vi "WLAN - TV - OPPO - RW - ReadTestVectorFile.vi"(5 "TV":string[][](array[string]), 7 "Measure Config":string[][](array[string])) -> (6 "Tv First Element":T2 {"Standard" items=["80211A/G/J/P OFDM", "80211B/G DSSS", "80211G DSSSOFDM", "80211N MIMOOFDM", "80211AC MIMOOFDM"]; "OFDM Data Rate (Mbps)" items=["6", "9", "12", "18", "24", "36", "48", "54"]; "80211n PLCP Frame Format" items=["Mixed Format", "Greenfield Format"]; "FEC Coding Type" items=["BCC", "LDPC"]; "DSSS Data Rate (Mbps)" items=["1", "2", "5.5 CCK", "5.5 PBCC", "11 CCK", "11 PBCC", "22", "33"]}, 10 "WLAN Measurement Settings":T3={"OFDM Advanced Controls(11ag)"={"OFDM Auto Compute Acquisition Length Enabled"=0, "OFDM Maximum Symbols Used"=0, "OFDM Time Tracking Enabled"=0, "OFDM Channel Tracking Enabled"=0, "OFDM Amplitude Tracking Enabled"=1, "OFDM CFO Estimation Method"=0, "OFDM Phase Tracking Method"=0, "OFDM Header Detection Enabled"=0, "OFDM MAC FCS Check Enabled"=0, "#Avg"=10, "#Iterations"=10}, "DSSS Demod Parameters"={"DSSS Auto Compute Acquisition Length Enabled"=0, "DSSS Equalization Enabled"=0, "DSSS Header Detection Enabled"=0, "DSSS MAC FCS Check Enabled"=0, "DSSS Measurement Start Location"=0, "DSSS Phase Tracking Method"=0, "DSSS Maximum Chips Used"=0, "DSSS Reference Pulse Shaping Filter"=0, "DSSS Reference Pulse Shaping Filter Coefficient"=0.0, "# Avg"=1024, "# Iterations"=1024, "DSSS Power Ramp Enabled"=0}, "OFDM Advanced Controls (11n)"={"OFDM Auto Compute Acquisition Length Enabled"=0, "OFDM Maximum Symbols Used"=0, "OFDM Time Tracking Enabled"=0, "OFDM Channel Tracking Enabled"=0, "OFDM Amplitude Tracking Enabled"=1, "OFDM CFO Estimation Method"=0, "OFDM Phase Tracking Method"=0, "OFDM Header Detection Enabled"=0, "OFDM MAC FCS Check Enabled"=0, "#Avg"=10, "#Iterations"=10}, "OFDM Advanced Controls(11ac)"={"OFDM Auto Compute Acquisition Length Enabled"=0, "OFDM Maximum Symbols Used"=0, "OFDM Time Tracking Enabled"=1, "OFDM Channel Tracking Enabled"=0, "OFDM Amplitude Tracking Enabled"=0, "OFDM CFO Estimation Method"=0, "OFDM Phase Tracking Method"=0, "OFDM Header Detection Enabled"=0, "OFDM MAC FCS Check Enabled"=0, "#Avg"=10, "#Iterations"=10}} {"OFDM Advanced Controls(11ac)"."OFDM Phase Tracking Method" items=["Standard", "Instantaneous", "None", "Standard with Cubic Spline Fit"]; "OFDM Advanced Controls(11ac)"."OFDM CFO Estimation Method" items=["Preamble Only", "Preamble and Data"]; "OFDM Advanced Controls(11ac)"."OFDM Channel Tracking Enabled" items=["False", "True"]; "OFDM Advanced Controls(11ac)"."OFDM Amplitude Tracking Enabled" items=["False", "True"]; "OFDM Advanced Controls(11ac)"."OFDM Time Tracking Enabled" items=["True"=1, "False"=0]; "OFDM Advanced Controls(11ac)"."OFDM Auto Compute Acquisition Length Enabled" items=["False", "True"]; "OFDM Advanced Controls(11ac)"."OFDM MAC FCS Check Enabled" items=["False", "True"]; "OFDM Advanced Controls(11ac)"."OFDM Header Detection Enabled" items=["False", "True"]; "OFDM Advanced Controls (11n)"."OFDM Phase Tracking Method" items=["Standard", "Instantaneous", "None", "Standard with Cubic Spline Fit"]; "OFDM Advanced Controls (11n)"."OFDM CFO Estimation Method" items=["Preamble Only", "Preamble and Data"]; "OFDM Advanced Controls (11n)"."OFDM Channel Tracking Enabled" items=["False", "True"]; "OFDM Advanced Controls (11n)"."OFDM Amplitude Tracking Enabled" items=["False", "True"]; "OFDM Advanced Controls (11n)"."OFDM Time Tracking Enabled" items=["True"=1, "False"=0]; "OFDM Advanced Controls (11n)"."OFDM Auto Compute Acquisition Length Enabled" items=["False", "True"]; "OFDM Advanced Controls (11n)"."OFDM MAC FCS Check Enabled" items=["False", "True"]; "OFDM Advanced Controls (11n)"."OFDM Header Detection Enabled" items=["False", "True"]; "DSSS Demod Parameters"."DSSS Power Ramp Enabled" items=["False", "True"]; "DSSS Demod Parameters"."DSSS Auto Compute Acquisition Length Enabled" items=["False", "True"]; "DSSS Demod Parameters"."DSSS Phase Tracking Method" items=["Standard", "Instantaneous"]; "DSSS Demod Parameters"."DSSS Equalization Enabled" items=["False", "True"]; "DSSS Demod Parameters"."DSSS Reference Pulse Shaping Filter" items=["Rectangular", "Raised Cosine", "Root Raised Cosine", "Gaussian"]; "DSSS Demod Parameters"."DSSS MAC FCS Check Enabled" items=["False", "True"]; "DSSS Demod Parameters"."DSSS Header Detection Enabled" items=["False", "True"]; "OFDM Advanced Controls(11ag)"."OFDM Phase Tracking Method" items=["Standard", "Instantaneous", "None", "Standard with Cubic Spline Fit"]; "OFDM Advanced Controls(11ag)"."OFDM CFO Estimation Method" items=["Preamble Only", "Preamble and Data"]; "OFDM Advanced Controls(11ag)"."OFDM Channel Tracking Enabled" items=["False", "True"]; "OFDM Advanced Controls(11ag)"."OFDM Amplitude Tracking Enabled" items=["False", "True"]; "OFDM Advanced Controls(11ag)"."OFDM Time Tracking Enabled" items=["True"=1, "False"=0]; "OFDM Advanced Controls(11ag)"."OFDM Auto Compute Acquisition Length Enabled" items=["False", "True"]; "OFDM Advanced Controls(11ag)"."OFDM MAC FCS Check Enabled" items=["False", "True"]; "OFDM Advanced Controls(11ag)"."OFDM Header Detection Enabled" items=["False", "True"]}, 14 "Cluster":T6)   [LabVIEW 2012]
uses:
  Includes/WLAN - TV - RW - INC - TV_DataType_Cluster.ctl
  Includes/WLAN - TV - RW - INC - Tx_Measurement_Cluster.ctl
  Includes/WLAN - TV - RW - INC - TV_OFDM Demod.ctl
  Includes/WLAN - TV - RW - INC - TV_DSSS Demod.ctl
  Includes/WLAN - TV - RW - INC - Tx_Measurement_Cluster(string).ctl
  Includes/WLAN - TV - RW - INC - Tx_Meas_Settings_OFDM_String.ctl
  Includes/WLAN - TV - RW - INC - Tx_Meas_Settings_DSSS_String.ctl
  Includes/WLAN - TV - RW - INC - TV_Parameters.ctl
panel:
  out "element":string
  in  "Tab Control":T1(tab)
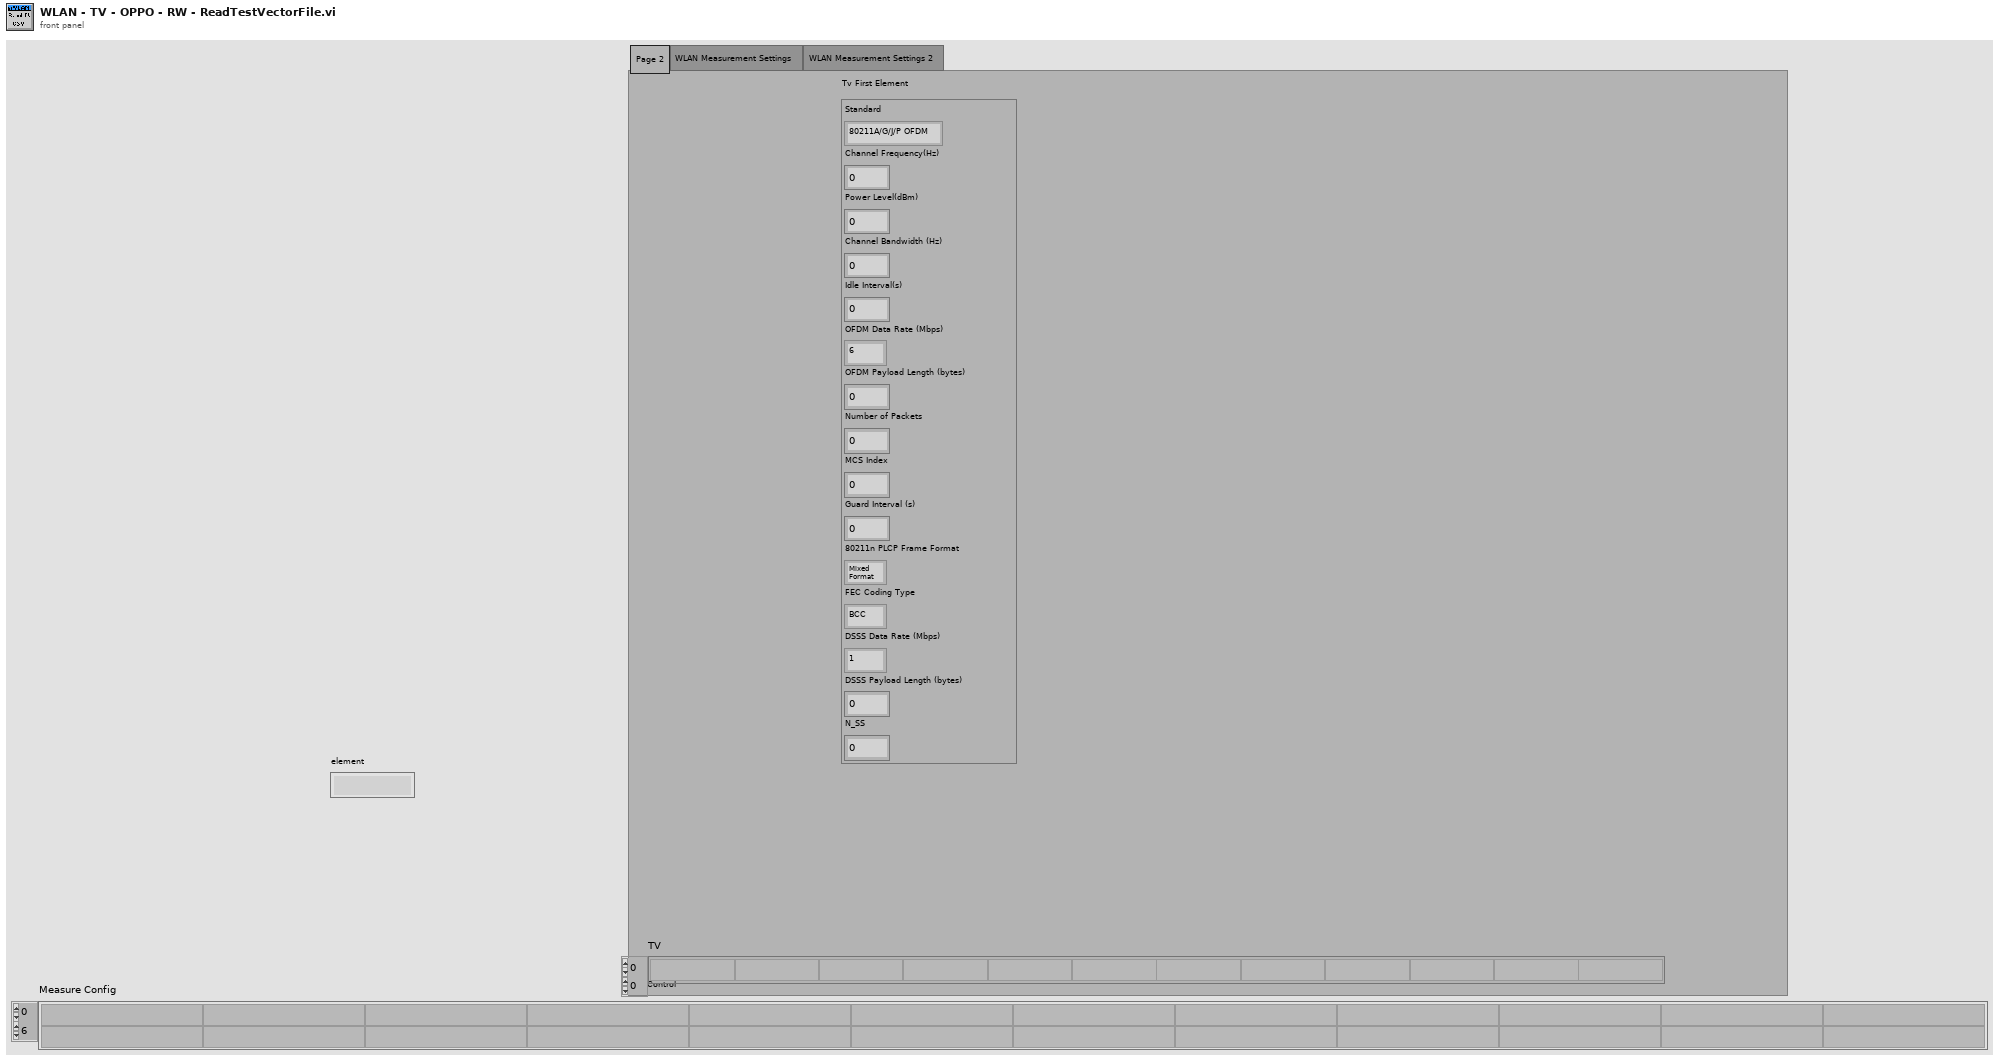
[diagram p1: front panel]
types:
  T1 = enum32{"Page 2", "WLAN Measurement Settings", "WLAN Measurement Settings 2"}
  T2 = typedef "WLAN - TV - RW - INC - TV_DataType_Cluster.ctl" = cluster{"Standard":i32, "Channel Frequency(Hz)":dbl, "Power Level(dBm)":dbl, "Channel Bandwidth (Hz)":dbl, "Idle Interval(s)":dbl, "OFDM Data Rate (Mbps)":i32, "OFDM Payload Length (bytes)":i32, "Number of Packets":i32, "MCS Index":i32, "Guard Interval (s)":dbl, "80211n PLCP Frame Format":i32, "FEC Coding Type":i32, "DSSS Data Rate (Mbps)":i32, "DSSS Payload Length (bytes)":i32, "N_SS":i32}
  T3 = typedef "WLAN - TV - RW - INC - Tx_Measurement_Cluster.ctl" = cluster{"OFDM Advanced Controls(11ag)":T4, "DSSS Demod Parameters":T5, "OFDM Advanced Controls (11n)":T4, "OFDM Advanced Controls(11ac)":cluster{"OFDM Auto Compute Acquisition Length Enabled":i32, "OFDM Maximum Symbols Used":i32, "OFDM Time Tracking Enabled":i32, "OFDM Channel Tracking Enabled":i32, "OFDM Amplitude Tracking Enabled":i32, "OFDM CFO Estimation Method":i32, "OFDM Phase Tracking Method":i32, "OFDM Header Detection Enabled":i32, "OFDM MAC FCS Check Enabled":i32, "#Avg":i32, "#Iterations":i32}}
  T4 = typedef "WLAN - TV - RW - INC - TV_OFDM Demod.ctl" = cluster{"OFDM Auto Compute Acquisition Length Enabled":i32, "OFDM Maximum Symbols Used":i32, "OFDM Time Tracking Enabled":i32, "OFDM Channel Tracking Enabled":i32, "OFDM Amplitude Tracking Enabled":i32, "OFDM CFO Estimation Method":i32, "OFDM Phase Tracking Method":i32, "OFDM Header Detection Enabled":i32, "OFDM MAC FCS Check Enabled":i32, "#Avg":i32, "#Iterations":i32}
  T5 = typedef "WLAN - TV - RW - INC - TV_DSSS Demod.ctl" = cluster{"DSSS Auto Compute Acquisition Length Enabled":i32, "DSSS Equalization Enabled":i32, "DSSS Header Detection Enabled":i32, "DSSS MAC FCS Check Enabled":i32, "DSSS Measurement Start Location":i32, "DSSS Phase Tracking Method":i32, "DSSS Maximum Chips Used":i32, "DSSS Reference Pulse Shaping Filter":i32, "DSSS Reference Pulse Shaping Filter Coefficient":dbl, "# Avg":i32, "# Iterations":i32, "DSSS Power Ramp Enabled":i32}
  T6 = typedef "WLAN - TV - RW - INC - Tx_Measurement_Cluster(string).ctl" = cluster{"OFDM Measurement Settings(11a)":T7, "TV Paramaters(11b)":T8, "OFDM Measurement Settings(11n) ":T7, "OFDM Measurement Settings(11ac) ":T7}
  T7 = typedef "WLAN - TV - RW - INC - Tx_Meas_Settings_OFDM_String.ctl" = cluster{"OFDM Auto Compute Acquisition Length Enabled":string, "OFDM Maximum Symbols Used":string, "OFDM Time Tracking Enabled":string, "OFDM Channel Tracking Enabled":string, "OFDM Amplitude Tracking Enabled":string, "OFDM CFO Estimation Method":string, "OFDM Phase Tracking Method":string, "OFDM Header Detection Enabled":string, "OFDM MAC FCS Check Enabled":string, "#Avg":string, "#Iterations":string}
  T8 = typedef "WLAN - TV - RW - INC - Tx_Meas_Settings_DSSS_String.ctl" = cluster{"DSSS Auto Compute Acquisition Length Enabled":string, "DSSS Equalization Enabled":string, "DSSS Header Detection Enabled":string, "DSSS MAC FCS Check Enabled":string, "DSSS Measurement Start Location":string, "DSSS Phase Tracking Method":string, "DSSS Maximum Chips Used":string, "DSSS Reference Pulse Shaping Filter":string, "DSSS Reference Pulse Shaping Filter Coefficient":string, "#Avg":string, "#Iterations":string, "DSSS Ramp Enabled ":string}
  T9 = typedef "WLAN - TV - RW - INC - TV_Parameters.ctl" = cluster{"Standard ":string, "Channel Frequency(Hz)":string, "Power Level(dBm)":string, "Channel Bandwidth (Hz)":string, "Idle Interval (s)":string, "OFDM Data Rate (Mbps)":string, "OFDM Payload Length (bytes)":string, "MCS Index":string, "Guard Interval (s)":string, "80211n PLCP Frame Format":string, "FEC Coding Type":string, "DSSS Data Rate (Mbps)":string, "DSSS Payload Length (bytes)":string, "#Packets":string, "N_SS":string}
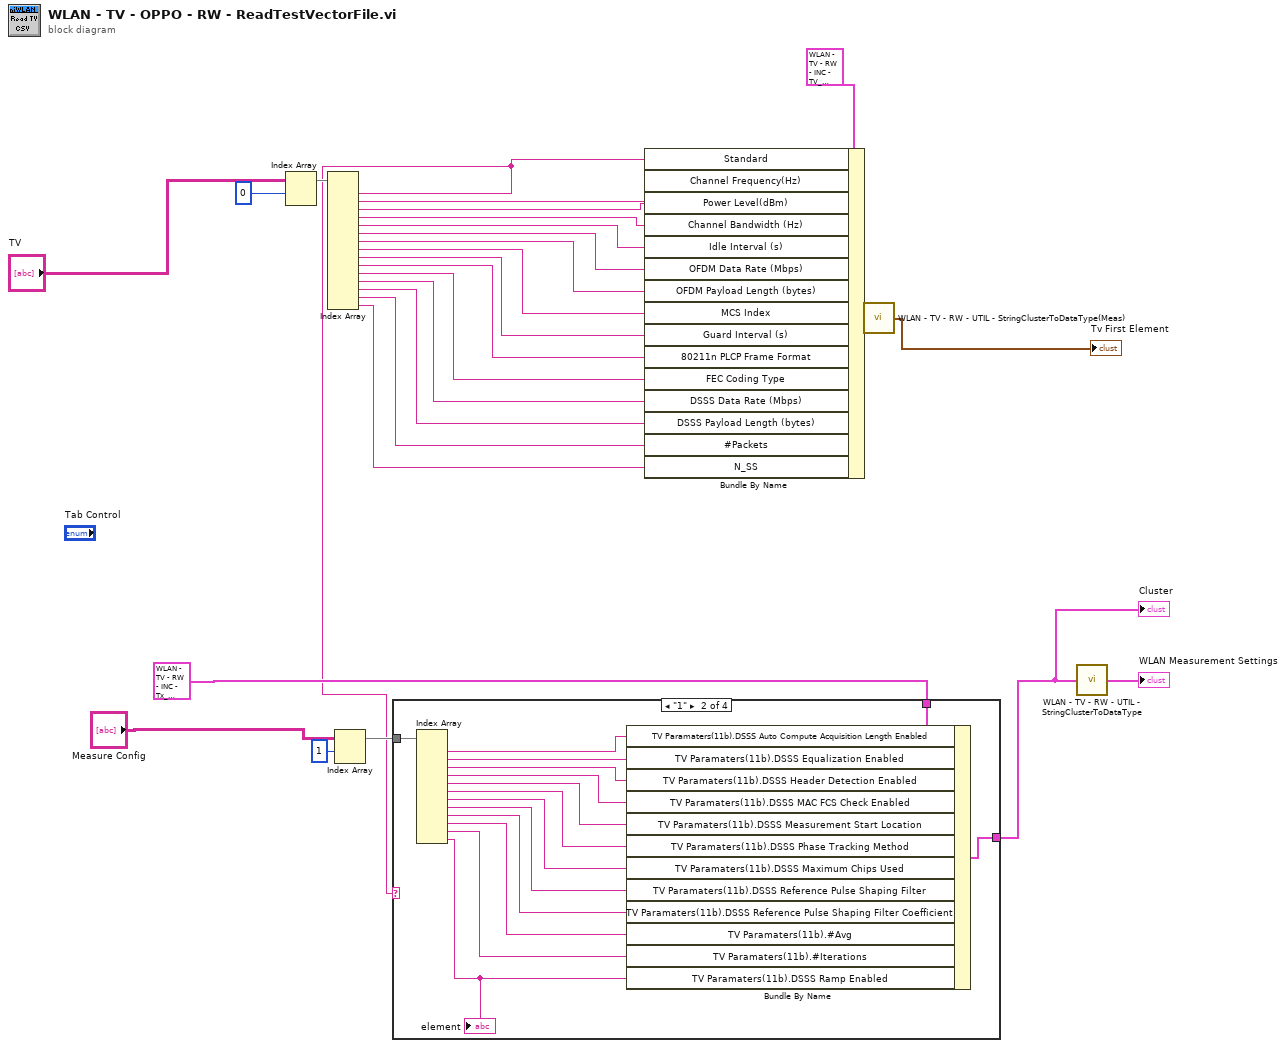
[diagram p0: block diagram]
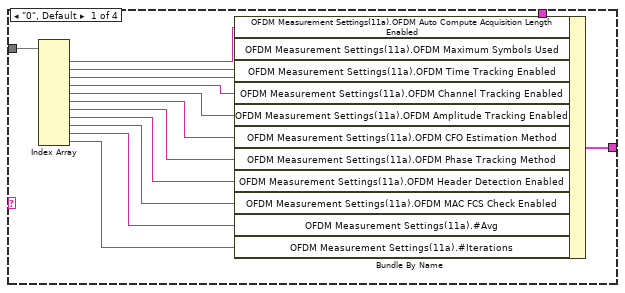
[diagram p2: hidden frame]
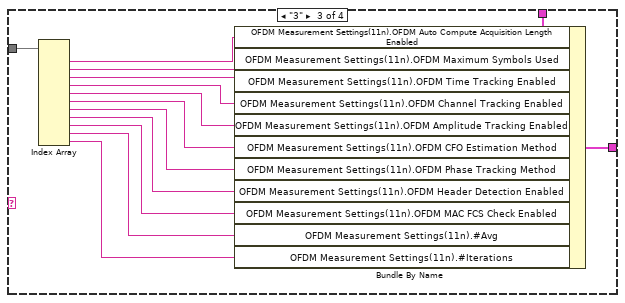
[diagram p3: hidden frame]
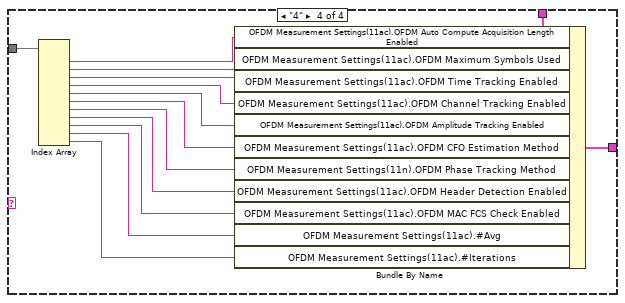
[diagram p4: hidden frame]
diagram:
  n1 = Index Array(array="TV", index (row)=0 ("x")) -> (element=w7:string[])  [unwired: 1 in]
  n2 = Index Array(array=w7) -> (element #1=w2:string, element #2=w21:string, element #3=w20:string, element #4=w19:string, element #5=w18:string, element #6=w17:string, element #7=w16:string, element #8=w15:string, element #9=w14:string, element #10=w13:string, element #11=w12:string, element #12=w11:string, element #13=w10:string, element #14=w9:string, element #15=w6:string)  [unwired: 15 in]
  n3 = Index Array(array="Measure Config", index (row)=1) -> (element=w5:string[])  [unwired: 1 in]
  n4 = case shown="\"1\"" w2 {
    tunnel: w5 -> [w41 w44 w70 w84]
    tunnel: T6 {"OFDM Measurement Settings(11a)"={"OFDM Auto Compute Acquisition Length Enabled"="", "OFDM Maximum Symbols Used"="", "OFDM Time Tracking Enabled"="", "OFDM Channel Tracking Enabled"="", "OFDM Amplitude Tracking Enabled"="", "OFDM CFO Estimation Method"="", "OFDM Phase Tracking Method"="", "OFDM Header Detection Enabled"="", "OFDM MAC FCS Check Enabled"="", "#Avg"="", "#Iterations"=""}, "TV Paramaters(11b)"={"DSSS Auto Compute Acquisition Length Enabled"="", "DSSS Equalization Enabled"="", "DSSS Header Detection Enabled"="", "DSSS MAC FCS Check Enabled"="", "DSSS Measurement Start Location"="", "DSSS Phase Tracking Method"="", "DSSS Maximum Chips Used"="", "DSSS Reference Pulse Shaping Filter"="", "DSSS Reference Pulse Shaping Filter Coefficient"="", "#Avg"="", "#Iterations"="", "DSSS Ramp Enabled "=""}, "OFDM Measurement Settings(11n) "={"OFDM Auto Compute Acquisition Length Enabled"="", "OFDM Maximum Symbols Used"="", "OFDM Time Tracking Enabled"="", "OFDM Channel Tracking Enabled"="", "OFDM Amplitude Tracking Enabled"="", "OFDM CFO Estimation Method"="", "OFDM Phase Tracking Method"="", "OFDM Header Detection Enabled"="", "OFDM MAC FCS Check Enabled"="", "#Avg"="", "#Iterations"=""}, "OFDM Measurement Settings(11ac) "={"OFDM Auto Compute Acquisition Length Enabled"="", "OFDM Maximum Symbols Used"="", "OFDM Time Tracking Enabled"="", "OFDM Channel Tracking Enabled"="", "OFDM Amplitude Tracking Enabled"="", "OFDM CFO Estimation Method"="", "OFDM Phase Tracking Method"="", "OFDM Header Detection Enabled"="", "OFDM MAC FCS Check Enabled"="", "#Avg"="", "#Iterations"=""}} ("Cluster") -> [w40 w43 w69 w83]
    tunnel: [w34 w42 w63 w77] -> w25
    frame "0", Default {
      n5 = Index Array(array=w41) -> (element #1=w39:string, element #2=w38:string, element #3=w37:string, element #4=w36:string, element #5=w35:string, element #6=w33:string, element #7=w32:string, element #8=w31:string, element #9=w30:string, element #10=w29:string, element #11=w28:string)  [unwired: 11 in]
      n6 = Bundle By Name(cluster=w40, "OFDM Measurement Settings(11a).OFDM Auto Compute Acquisition Length Enabled"=w39, "OFDM Measurement Settings(11a).OFDM Maximum Symbols Used"=w38, "OFDM Measurement Settings(11a).OFDM Time Tracking Enabled"=w37, "OFDM Measurement Settings(11a).OFDM Channel Tracking Enabled"=w36, "OFDM Measurement Settings(11a).OFDM Amplitude Tracking Enabled"=w35, "OFDM Measurement Settings(11a).OFDM CFO Estimation Method"=w33, "OFDM Measurement Settings(11a).OFDM Phase Tracking Method"=w32, "OFDM Measurement Settings(11a).OFDM Header Detection Enabled"=w31, "OFDM Measurement Settings(11a).OFDM MAC FCS Check Enabled"=w30, "OFDM Measurement Settings(11a).#Avg"=w29, "OFDM Measurement Settings(11a).#Iterations"=w28) -> (w34:T6)
    }
    frame "1" {
      n7 = Index Array(array=w44) -> (element #1=w56:string, element #2=w55:string, element #3=w54:string, element #4=w53:string, element #5=w52:string, element #6=w51:string, element #7=w50:string, element #8=w49:string, element #9=w48:string, element #10=w47:string, element #11=w46:string, element #12=w45:string)  [unwired: 12 in]
      "element" <- w45
      n8 = Bundle By Name(cluster=w43, "TV Paramaters(11b).DSSS Auto Compute Acquisition Length Enabled"=w56, "TV Paramaters(11b).DSSS Equalization Enabled"=w55, "TV Paramaters(11b).DSSS Header Detection Enabled"=w54, "TV Paramaters(11b).DSSS MAC FCS Check Enabled"=w53, "TV Paramaters(11b).DSSS Measurement Start Location"=w52, "TV Paramaters(11b).DSSS Phase Tracking Method"=w51, "TV Paramaters(11b).DSSS Maximum Chips Used"=w50, "TV Paramaters(11b).DSSS Reference Pulse Shaping Filter"=w49, "TV Paramaters(11b).DSSS Reference Pulse Shaping Filter Coefficient"=w48, "TV Paramaters(11b).#Avg"=w47, "TV Paramaters(11b).#Iterations"=w46, "TV Paramaters(11b).DSSS Ramp Enabled"=w45) -> (w42:T6)
    }
    frame "3" {
      n9 = Index Array(array=w70) -> (element #1=w68:string, element #2=w67:string, element #3=w66:string, element #4=w65:string, element #5=w64:string, element #6=w62:string, element #7=w61:string, element #8=w60:string, element #9=w59:string, element #10=w58:string, element #11=w57:string)  [unwired: 11 in]
      n10 = Bundle By Name(cluster=w69, "OFDM Measurement Settings(11n).OFDM Auto Compute Acquisition Length Enabled"=w68, "OFDM Measurement Settings(11n).OFDM Maximum Symbols Used"=w67, "OFDM Measurement Settings(11n).OFDM Time Tracking Enabled"=w66, "OFDM Measurement Settings(11n).OFDM Channel Tracking Enabled"=w65, "OFDM Measurement Settings(11n).OFDM Amplitude Tracking Enabled"=w64, "OFDM Measurement Settings(11n).OFDM CFO Estimation Method"=w62, "OFDM Measurement Settings(11n).OFDM Phase Tracking Method"=w61, "OFDM Measurement Settings(11n).OFDM Header Detection Enabled"=w60, "OFDM Measurement Settings(11n).OFDM MAC FCS Check Enabled"=w59, "OFDM Measurement Settings(11n).#Avg"=w58, "OFDM Measurement Settings(11n).#Iterations"=w57) -> (w63:T6)
    }
    frame "4" {
      n11 = Index Array(array=w84) -> (element #1=w82:string, element #2=w81:string, element #3=w80:string, element #4=w79:string, element #5=w78:string, element #6=w76:string, element #7=w75:string, element #8=w74:string, element #9=w73:string, element #10=w72:string, element #11=w71:string)  [unwired: 11 in]
      n12 = Bundle By Name(cluster=w83, "OFDM Measurement Settings(11ac).OFDM Auto Compute Acquisition Length Enabled"=w82, "OFDM Measurement Settings(11ac).OFDM Maximum Symbols Used"=w81, "OFDM Measurement Settings(11ac).OFDM Time Tracking Enabled"=w80, "OFDM Measurement Settings(11ac).OFDM Channel Tracking Enabled"=w79, "OFDM Measurement Settings(11ac).OFDM Amplitude Tracking Enabled"=w78, "OFDM Measurement Settings(11ac).OFDM CFO Estimation Method"=w76, "OFDM Measurement Settings(11n).OFDM Phase Tracking Method"=w75, "OFDM Measurement Settings(11ac).OFDM Header Detection Enabled"=w74, "OFDM Measurement Settings(11ac).OFDM MAC FCS Check Enabled"=w73, "OFDM Measurement Settings(11ac).#Avg"=w72, "OFDM Measurement Settings(11ac).#Iterations"=w71) -> (w77:T6)
    }
  }
  "Cluster" <- w25
  n13 = Bundle By Name(cluster=T9 {"Standard "="", "Channel Frequency(Hz)"="", "Power Level(dBm)"="", "Channel Bandwidth (Hz)"="", "Idle Interval (s)"="", "OFDM Data Rate (Mbps)"="", "OFDM Payload Length (bytes)"="", "MCS Index"="", "Guard Interval (s)"="", "80211n PLCP Frame Format"="", "FEC Coding Type"="", "DSSS Data Rate (Mbps)"="", "DSSS Payload Length (bytes)"="", "#Packets"="", "N_SS"=""} ("TV Paramaters"), "Standard"=w2, "Channel Frequency(Hz)"=w21, "Power Level(dBm)"=w20, "Channel Bandwidth (Hz)"=w19, "Idle Interval (s)"=w18, "OFDM Data Rate (Mbps)"=w17, "OFDM Payload Length (bytes)"=w16, "MCS Index"=w15, "Guard Interval (s)"=w14, "80211n PLCP Frame Format"=w13, "FEC Coding Type"=w12, "DSSS Data Rate (Mbps)"=w11, "DSSS Payload Length (bytes)"=w10, "#Packets"=w9, "N_SS"=w6) -> (w8:T9)
  n14 = call "WLAN - TV - RW - UTIL - StringClusterToDataType(Meas).vi"("TV Paramaters(String)"=w8) -> ("TV Parameters(DataType)"=→"Tv First Element":T2)  [unwired: 14 in]
  n15 = call "WLAN - TV - RW - UTIL - StringClusterToDataType.vi"("TV Paramaters(String)"=w25) -> ("WLAN Measurement Settings"=→"WLAN Measurement Settings":T3)  [unwired: 14 in]
